vi "FlatToRichsift_proxy_v1_ChannelBitFieldElement.vi"(5 "OutputClusterType":T1, 11 "InputCluster":T2) -> (3 "OutputCluster":T1)   [LabVIEW 2024, in "SiftProxy_client.lvlib"]
uses:
  sift_proxy_v1_ChannelBitFieldElement_Flat.ctl
  sift_proxy_v1_ChannelBitFieldElement.ctl
  SiftProxy_client.lvlib
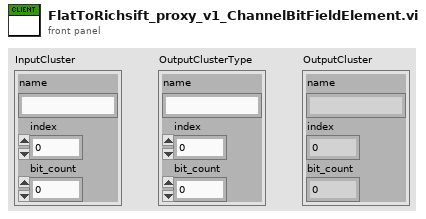
[diagram p1: front panel]
types:
  T1 = typedef "SiftProxy_client.lvlib/sift_proxy_v1_ChannelBitFieldElement.ctl" = cluster{"name":string, "index":i32, "bit_count":u32}
  T2 = typedef "SiftProxy_client.lvlib/sift_proxy_v1_ChannelBitFieldElement_Flat.ctl" = cluster{"name":string, "index":i32, "bit_count":u32}
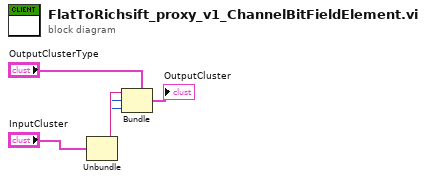
[diagram p0: block diagram]
diagram:
  n1 = Unbundle "Unbundle"("InputCluster") -> ("name"=w3:string, "index"=w2:i32, "bit_count"=w1:u32)
  n2 = Bundle "Bundle"(cluster="OutputClusterType", "name"=w3, "index"=w2, "bit_count"=w1) -> (→"OutputCluster":T1)
